vi "Delete All But Current Folder Hierarchy.vi"(8 "error in":errorcluster, 10 "Item Tag":string, 11 "TreeControl in":refnum<vi>) -> (0 "error out":errorcluster, 2 "Deleted Folders":path[](array[path]), 3 "TreeControl out":refnum<vi>)   [LabVIEW 2013, in "LVTM.lvlib"]
uses:
  LVTM.lvlib
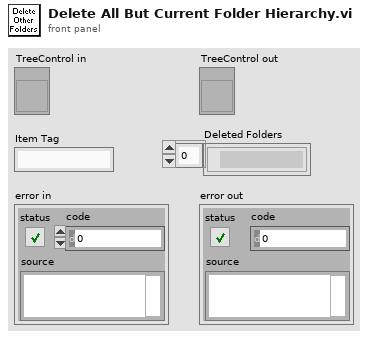
[diagram p1: front panel]
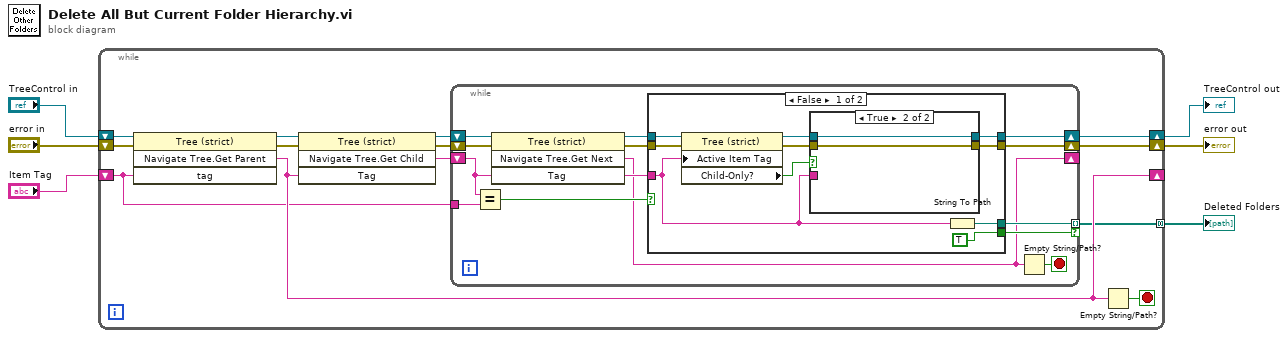
[diagram p0: block diagram]
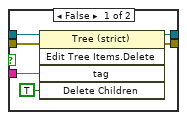
[diagram p2: hidden frame]
diagram:
  n1 = while {
    shift-right: [w13] -> w5
    shift-left: "TreeControl in" -> [w19]
    shift-right: [w10] -> _
    shift-left: "Item Tag" -> [w8]
    shift-right: [w12] -> w6
    shift-left: "error in" -> [w11]
    tunnel: [w7] -> w1 mode=concatenating
    stop <- w9 stop-if-true
    n2 = invoke class="Tree (strict)" method="Navigate Tree.Get Parent"(reference=w19, error in=w11, "tag"=w8) -> (reference out=w18:refnum<vi>, error out=w17:errorcluster, "Navigate Tree:Get Parent"=w10:string)  [unwired: 1 in, 1 out]
    n3 = invoke class="Tree (strict)" method="Navigate Tree.Get Child"(reference=w18, error in=w17, "Tag"=w10) -> (reference out=w16:refnum<vi>, error out=w15:errorcluster, "Navigate Tree:Get Child"=w14:string)  [unwired: 1 in, 1 out]
    n4 = while {
      tunnel: w8 -> [w32]
      shift-right: [w25] -> w12
      shift-left: w15 -> [w28]
      shift-right: [w24] -> w13
      shift-left: w16 -> [w30]
      shift-right: [w20] -> _
      shift-left: w14 -> [w23]
      tunnel: [w21] -> w7 mode=indexing if=w22
      stop <- w26 stop-if-true
      n5 = Equal?(x=w23, y=w32) -> (x = y?=w31:bool)
      n6 = invoke class="Tree (strict)" method="Navigate Tree.Get Next"(reference=w30, error in=w28, "Tag"=w23) -> (reference out=w29:refnum<vi>, error out=w27:errorcluster, "Navigate Tree:Get Next Item"=w20:string)  [unwired: 1 in, 1 out]
      n7 = case shown="False" w31 {
        tunnel: w29 -> [w38 w52]
        tunnel: w27 -> [w36 w51]
        tunnel: w23 -> [w34 _]
        tunnel: [w42 w52] -> w24
        tunnel: [w41 w51] -> w25
        tunnel: [TRUE ("Delete Children?") _] -> w22
        tunnel: [w39 _] -> w21
        frame False {
          n8 = property class="Tree (strict)"(reference=w38, error in=w36, "Active Item Tag"=w34) -> (reference out=w37:refnum<vi>, error out=w35:errorcluster, "Child-Only?"=w33:bool)
          n9 = case shown="True" w33 {
            tunnel: [w47 w50] -> w42
            tunnel: [w46 w49] -> w41
            tunnel: w37 -> [w45 w50]
            tunnel: w35 -> [w44 w49]
            tunnel: w34 -> [w43 _]
            frame False {
              n10 = invoke class="Tree (strict)" method="Edit Tree Items.Delete"(reference=w45, error in=w44, "tag"=w43, "Delete Children"=TRUE ("Delete Children?")) -> (reference out=w47:refnum<vi>, error out=w46:errorcluster)  [unwired: 1 in, 3 out]
            }
            frame True {
            }
          }
          n11 = String To Path(string=w34) -> (path=w39:path)
        }
        frame True {
        }
      }
      n12 = Empty String/Path?(string/path=w20) -> (empty?=w26:bool)
    }
    n13 = Empty String/Path?(string/path=w10) -> (empty?=w9:bool)
  }
  "error out" <- w6
  "TreeControl out" <- w5
  "Deleted Folders" <- w1
